vi "myRIO__TCP_constants_byteRange_messageType__checkRange.vi"(11 "input_byte":u8) -> (0 "output_selectResponse":bool, 1 "output_trial":bool, 2 "output_block":bool, 3 "output_messageType":bool, 4 "output_analogInput":bool, 5 "output_quit":bool, 7 "output_start":bool)   [LabVIEW 2014]
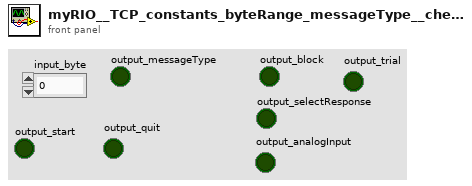
[diagram p1: front panel]
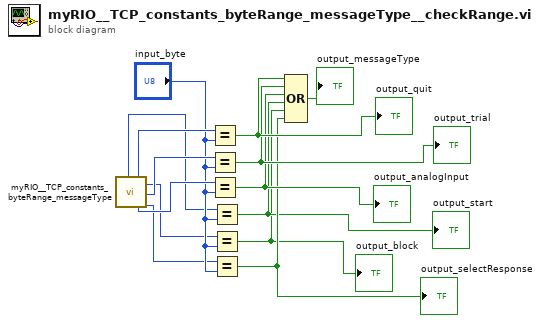
[diagram p0: block diagram]
diagram:
  n1 = call "myRIO__TCP_constants_byteRange_messageType.vi"() -> ("output_Start_byte"=w5:u8, "output_Quit_byte"=w10:u8, "output_analogInput_byte"=w8:u8, "output_Block_byte"=w3:u8, "output_Trial_byte"=w9:u8, "output_selectResponse_byte"=w4:u8)  [unwired: 8 in, 6 out]
  n2 = Equal?(x=w10, y="input_byte") -> (x = y?=w13:bool)
  "output_quit" <- w13
  n3 = Equal?(x=w9, y="input_byte") -> (x = y?=w12:bool)
  "output_trial" <- w12
  n4 = Equal?(x=w8, y="input_byte") -> (x = y?=w11:bool)
  "output_analogInput" <- w11
  n5 = Equal?(x=w5, y="input_byte") -> (x = y?=w2:bool)
  "output_start" <- w2
  n6 = Equal?(x=w3, y="input_byte") -> (x = y?=w1:bool)
  "output_block" <- w1
  n7 = Equal?(x=w4, y="input_byte") -> (x = y?=w6:bool)
  "output_selectResponse" <- w6
  n8 = Compound Arithmetic op=OR(w13, w12, w11, w2, w1, w6) -> (→"output_messageType":bool)
